vi "launch_wait.vi"(8 "error in (no error)":errorcluster, 9 "steps":variant, 10 "recipe_data in":variant, 11 "data":variant) -> (0 "error out":errorcluster)   [LabVIEW 2015, in "lv-recipe-machine.lvlib" / "example_01.lvlib"]
doc: "launch_wait.vi is an example that will launch three wait processes asynchronously, hi-jack their transition queues to point to itself, aggregate their output and provide a result via the recipe_machine transition queue."
uses:
  example_01.lvlib
  public/_controls/transition.ctl
  public/_controls/error.ctl
  _controls/steps_actions_data.ctl
  _controls/steps_actions.ctl
  public/_controls/vi_reference_type.ctl
  lv-recipe-machine.lvlib
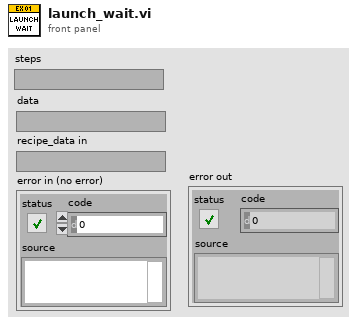
[diagram p1: front panel]
types:
  T1 = typedef "lv-recipe-machine.lvlib/vi_reference_type.ctl" = enum16{"<vi_reference_type>", "manual_action", "auto_step", "auto_criteria", "auto_transition", "auto_launcher", "<null>"}
  T2 = typedef "lv-recipe-machine.lvlib/error.ctl" = enum16{"<error>", "bad_command", "command_queue_timeout", "stop_notifier_timeout", "die_command_timeout", "not_in_manual_mode", "not_in_automatic_mode", "not_in_automatic_idle", "not_in_automatic_running", "not_in_automatic_paused", "automatic_step_not_found", "manual_action_not_found", "automatic_not_transition_vi", "transition_step_not_found", "unsupported_vi_type", "<null>"}
  T3 = typedef "lv-recipe-machine.lvlib/example_01.lvlib/steps_actions.ctl" = enum16{"<steps_actions>", "manual_random", "manual_comparison", "manual_wait", "auto_random", "auto_wait", "criteria_initialize", "criteria_count", "criteria_comparison", "transition_simple", "transition_count", "transition_comparison", "launch_wait", "<null>"}
  T4 = typedef "lv-recipe-machine.lvlib/example_01.lvlib/steps_actions_data.ctl" = cluster{"step_action":T3, "data":variant}
  T5 = typedef "lv-recipe-machine.lvlib/transition.ctl" = cluster{"next_index":i32, "data":variant, "recipe_data":variant, "error":errorcluster}
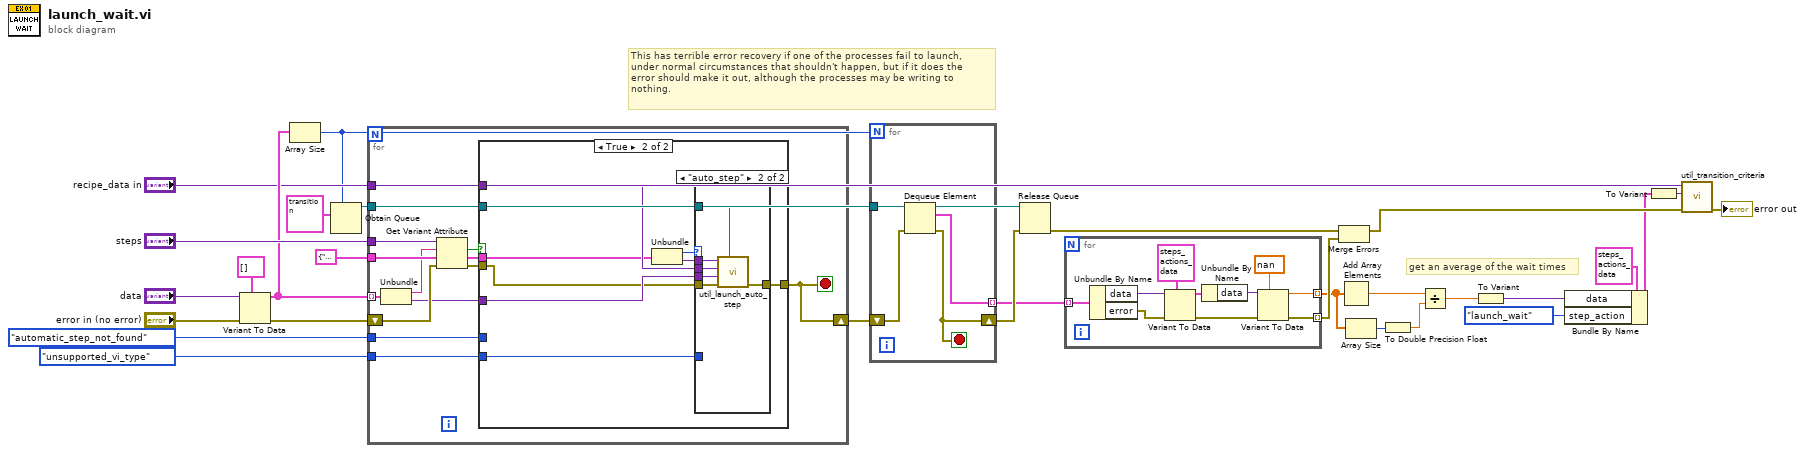
[diagram p0: block diagram]
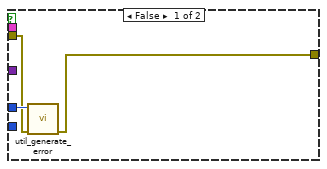
[diagram p2: hidden frame]
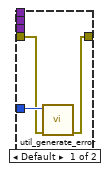
[diagram p3: hidden frame]
diagram:
  # "This has terrible error recovery if one of the processes fail to launch,\nunder normal circumstances that shouldn't happen, but if it does the\nerror should make it out, although the processes may be writing to\nnothing."
  # "get an average of the wait times"
  n1 = Variant To Data(error in="error in (no error)", type=cluster{"step":string, "data":variant}[] [], Variant="data") -> (data=w23:cluster{"step":string, "data":variant}[], error out=w26:errorcluster)
  n2 = Array Size(array=w23) -> (size(s)=w20:i32)
  n3 = Obtain Queue(max queue size (-1, unlimited)=w20, element data type=T5 {"next_index"=0, "data"=variant, "recipe_data"=variant, "error"={"status"=FALSE, "code"=0, "source"=""}} ("transition")) -> (queue out=w19:refnum<queue>)  [unwired: 3 in, 2 out]
  n4 = for {
    tunnel: w23 -> [w43] mode=indexing
    shift-right: [w32] -> w18
    shift-left: w26 -> [w44]
    tunnel: "steps" -> [w42]
    tunnel: cluster{"type":T1, "vi_reference":variant} {"type"=enum."<vi_reference_type>", "vi_reference"=variant} -> [w41]
    tunnel: error."automatic_step_not_found" ("error") -> [w37]
    tunnel: w19 -> [w36]
    tunnel: "recipe_data in" -> [w35]
    tunnel: error."unsupported_vi_type" ("error") -> [w31]
    stop <- w32 stop-if-true
    n5 = Unbundle(w43) -> ("step"=w34:string, "data"=w33:variant)
    n6 = Get Variant Attribute(Variant=w42, name=w34, default value (empty Variant)=w41, error in=w44) -> (found=w40:bool, value=w39:cluster{"type":T1, "vi_reference":variant}, error out=w38:errorcluster)  [unwired: 1 out]
    n7 = case shown="True" w40 {
      tunnel: w39 -> [_ w49]
      tunnel: w38 -> [w46 w48]
      tunnel: w37 -> [w47 _]
      tunnel: w36 -> [_ w56]
      tunnel: w35 -> [_ w55]
      tunnel: w33 -> [_ w54]
      tunnel: [w45 w53] -> w32
      tunnel: w31 -> [_ w50]
      frame False {
        n8 = call "util_generate_error.vi"("error in (no error)"=w46, "error"=w47) -> ("error out"=w45:errorcluster)  [unwired: 9 in]
      }
      frame True {
        n9 = Unbundle(w49) -> ("type"=w51:T1, "vi_reference"=w52:variant)
        n10 = case shown="\"auto_step\"" w51 {
          tunnel: w56 -> [_ w65]
          tunnel: w55 -> [_ w64]
          tunnel: w54 -> [_ w63]
          tunnel: [w57 w62] -> w53
          tunnel: w52 -> [_ w61]
          tunnel: w50 -> [w59 _]
          tunnel: w48 -> [w58 w60]
          frame Default {
            n11 = call "util_generate_error.vi"("error in (no error)"=w58, "error"=w59) -> ("error out"=w57:errorcluster)  [unwired: 9 in]
          }
          frame "auto_step" {
            n12 = call "util_launch_auto_step.vi"("transition_queue"=w65, "error in (no error)"=w60, "data"=w63, "recipe_data"=w64, "vi_reference"=w61) -> ("error out"=w62:errorcluster)  [unwired: 6 in]
          }
        }
      }
    }
  }
  n13 = for {
    N: w20 -> [_]
    tunnel: w19 -> [w69]
    shift-right: [w67] -> w17
    shift-left: w18 -> [w68]
    tunnel: [w66] -> w16 mode=indexing
    stop <- w67 stop-if-true
    n14 = Dequeue Element(queue=w69, error in (no error)=w68) -> (element=w66:T5, error out=w67:errorcluster)  [unwired: 1 in, 2 out]
  }
  n15 = Release Queue(queue=w19, error in (no error)=w17) -> (error out=w15:errorcluster)  [unwired: 1 in, 2 out]
  n16 = for {
    tunnel: w16 -> [w79] mode=indexing
    tunnel: [w77] -> w4 mode=indexing
    tunnel: [w76] -> w13 mode=indexing
    n17 = Unbundle By Name(w79) -> ("data"=w75:variant, "error"=w74:errorcluster)
    n18 = Variant To Data(error in=w74, type=T4 {"step_action"=enum."<steps_actions>", "data"=variant} ("step_data"), Variant=w75) -> (data=w71:T4, error out=w73:errorcluster)
    n19 = Unbundle By Name(w71) -> ("data"=w70:variant)
    n20 = Variant To Data(error in=w73, type=nan, Variant=w70) -> (data=w77:dbl, error out=w76:errorcluster)
  }
  n21 = Merge Errors(w15, w13) -> (w14:errorcluster)
  n22 = Add Array Elements(numeric array=w4) -> (sum=w11:dbl)
  n23 = Array Size(array=w4) -> (size(s)=w3:i32)
  n24 = To Double Precision Float(number=w3) -> (double precision float=w2:dbl)
  n25 = Divide(x=w11, y=w2) -> (x/y=w5:dbl)
  n26 = To Variant(anything=w5) -> (Variant=w10:variant)
  n27 = Bundle By Name(cluster=T4 {"step_action"=enum."<steps_actions>", "data"=variant}, "data"=w10, "step_action"=steps_actions."launch_wait") -> (w8:T4)
  n28 = To Variant(anything=w8) -> (Variant=w7:variant)
  n29 = call "util_transition_criteria.vi"("error in (no error)"=w14, "data"=w7, "recipe_data"="recipe_data in") -> ("error out"=→"error out":errorcluster)  [unwired: 8 in]
